vi "COD浓度全局变量.vi"() -> ()   [LabVIEW 2016, in "斯坦道CODMn.lvlib"]
panel:
  out "配置文件ini":string
  out "序列号:":string
  in  "VISA resource name":refnum<visa-resource-name>="COM4" caption="VISA资源名称"
  in  "基本量程":enum16{"10mg/L", "20mg/L"}(ring)
  in  "浓度 2":dbl
  in  "跨度液浓度":dbl
  in  "COD浓度（mg/L)":dbl
  # "跨度液浓度："
  # "标准液浓度（mg/L）："
  # "基本量程（20mL可选）："
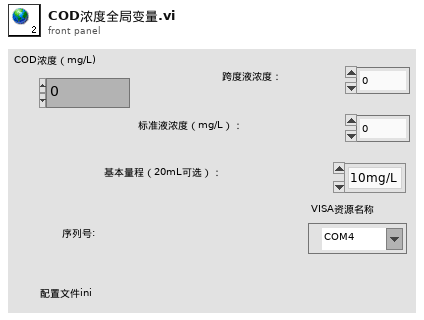
[diagram p1: front panel]
diagram:
